vi "StartWindowDrag.vi"(8 "error in":errorcluster, 11 "VI Ref (calling VI)":refnum<vi>) -> (0 "error out":errorcluster, 3 "dup VI Ref":refnum<vi>)   [LabVIEW 2025, in "UI_Library.lvlib" / "UI_Library.lvclass"]
doc: "Handle Windows SO user32.dll to obtain the window drag effect on a custom Control\nonly window SO"
uses:
  UI_Library.lvclass
  user32.dll
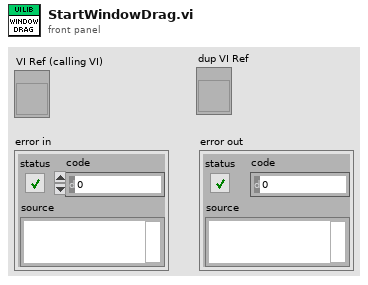
[diagram p1: front panel]
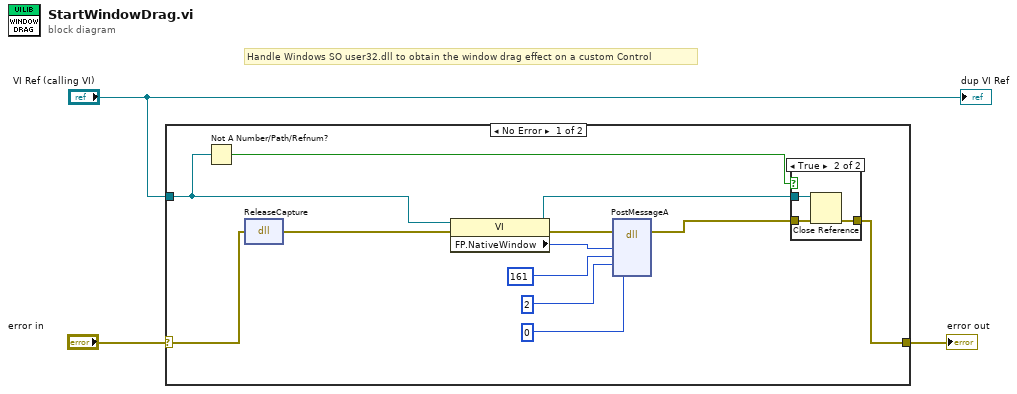
[diagram p0: block diagram]
diagram:
  # "Handle Windows SO user32.dll to obtain the window drag effect on a custom Control"
  n1 = case shown="No Error" "error in" {
    selector: "error in" -> [w15 w20]
    tunnel: "VI Ref (calling VI)" -> [w8 _]
    tunnel: [w4 w20] -> w3
    frame No Error {
      n2 = Not A Number/Path/Refnum?(number/path/refnum=w8) -> (NaN/Path/Refnum?=w7:bool)
      n3 = dll-call lib="user32.dll" fn="ReleaseCapture"(error in=w15) -> (error out=w14:errorcluster)  [unwired: 3 in, 1 out]
      n4 = property class="VI"(reference=w8, error in=w14) -> (reference out=w6:refnum<vi>, error out=w13:errorcluster, "FP.NativeWindow"=w12:u64)
      n5 = dll-call lib="user32.dll" fn="PostMessageA"(error in=w13, "hWnd"=w12, "Msg"=161, "wParam"=2, "lParam"=0) -> (error out=w5:errorcluster)  [unwired: 7 in, 1 out]
      n6 = case shown="True" w7 {
        tunnel: w6 -> [_ w19]
        tunnel: w5 -> [w16 w18]
        tunnel: [w16 w17] -> w4
        frame False {
        }
        frame True {
          n7 = Close Reference(reference=w19, error in (no error)=w18) -> (error out=w17:errorcluster)
        }
      }
    }
    frame Error {
    }
  }
  "error out" <- w3
  "dup VI Ref" <- "VI Ref (calling VI)"
